vi "Save Error Logs.vi"(6 "Finish?":bool, 7 "T: no error Save":bool, 8 "error in (no error)":errorcluster, 10 "States In":string, 11 "FileName":string="Process") -> (0 "error out":errorcluster)   [LabVIEW 2021]
uses:
  TopPath/TopPath.lvlib
  <vilib>/Utility/file.llb/Write Delimited Spreadsheet (string).vi
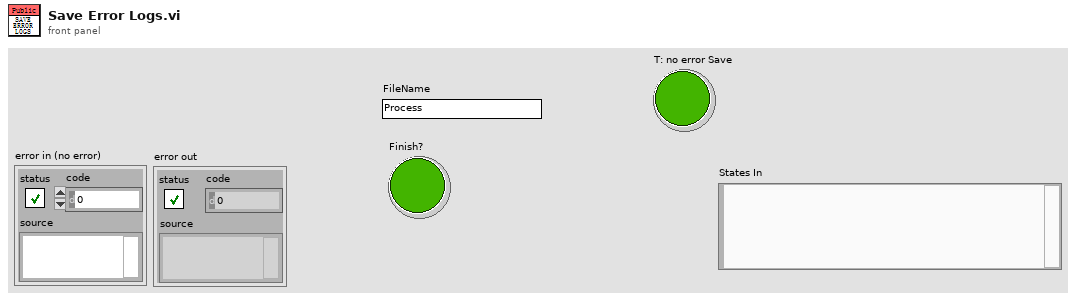
[diagram p1: front panel]
types:
  T1 = typedef "TopPath.lvlib/Top Path.ctl" = cluster{"LV Source":path, "FilePath":path, "Data":path}
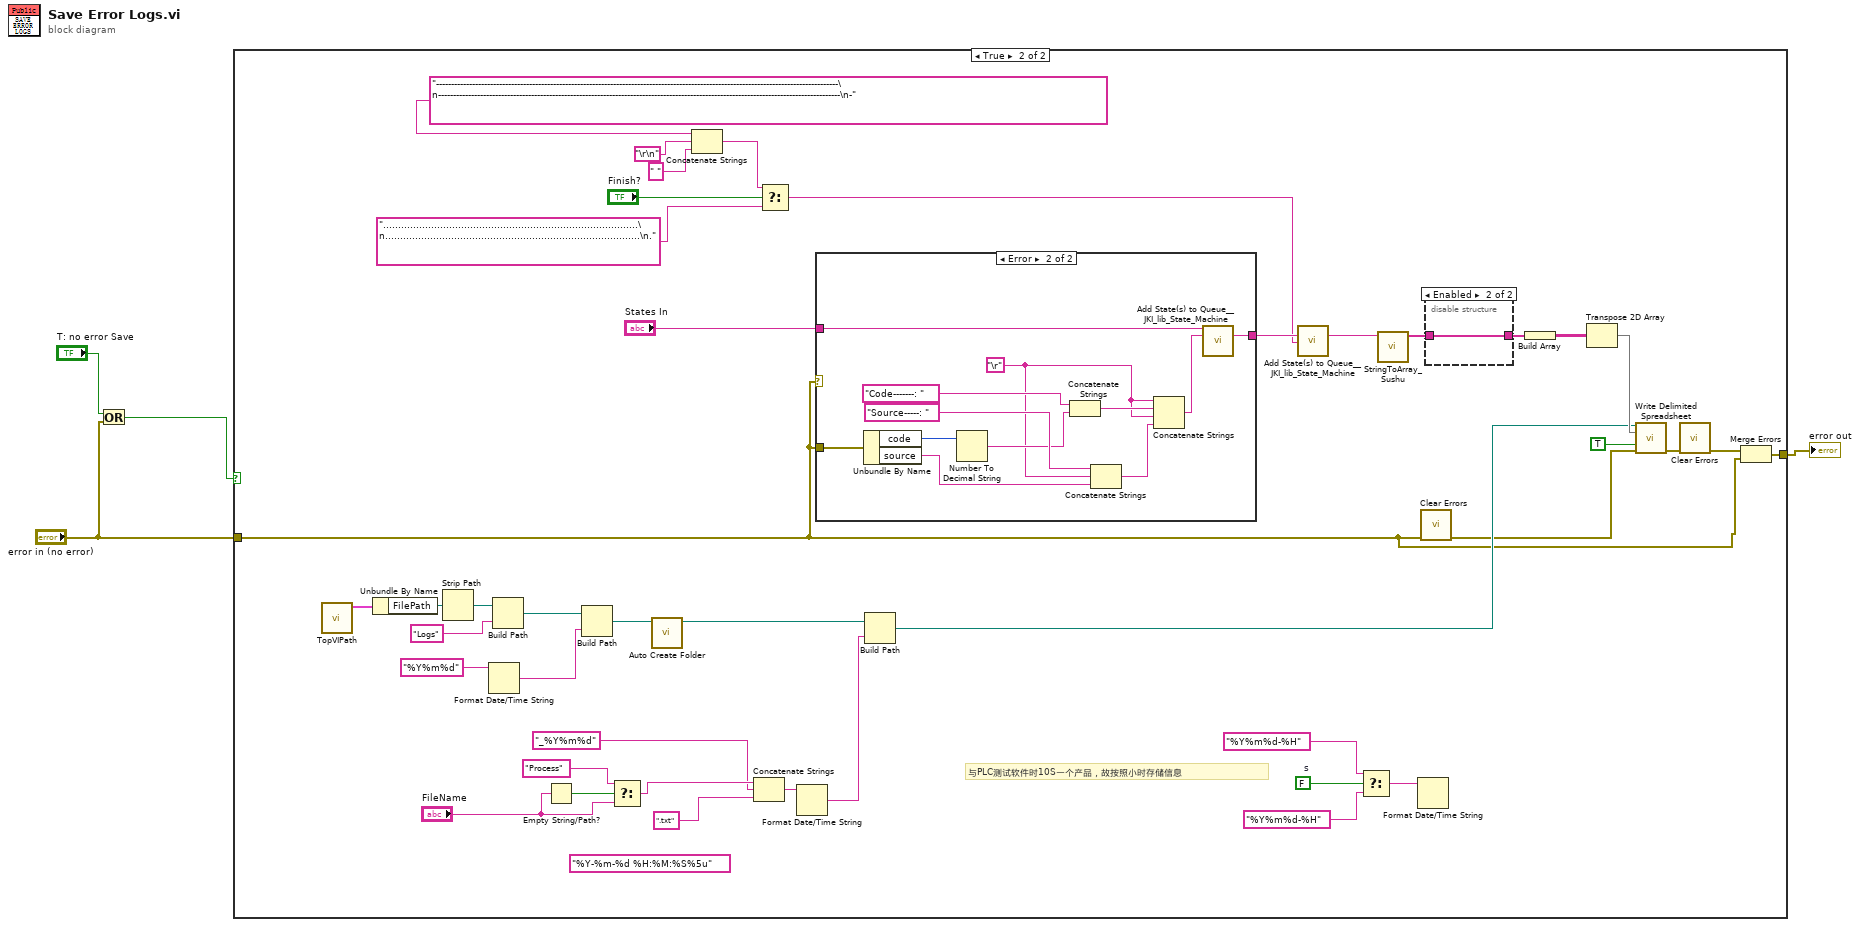
[diagram p0: block diagram]
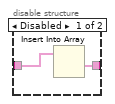
[diagram p4: hidden frame]
diagram:
  n1 = Or(x="T: no error Save", y="error in (no error)") -> (x .or. y?=w1:bool)
  n2 = case shown="True" w1 {
    tunnel: "error in (no error)" -> [w5 w7]
    tunnel: [w5 w9] -> w4
    frame False {
    }
    frame True {
      w11 = FALSE  # s
      (unwired) "%Y-%m-%d %H:%M:%S%5u" ("time format string (%c)")
      # "与PLC测试软件时10S一个产品，故按照小时存储信息"
      n3 = call "TopVIPath.vi"() -> ("TopPath"=w33:T1)  [unwired: 10 in, 1 out]
      n4 = Unbundle By Name(w33) -> ("FilePath"=w34:path)
      n5 = Strip Path(path=w34) -> (stripped path=w23:path)  [unwired: 1 out]
      n6 = Format Date/Time String(time format string (%c)="%Y%m%d") -> (date/time string=w12:string)  [unwired: 2 in]
      n7 = Build Path(base path=w23, name or relative path="Logs") -> (appended path=w15:path)
      n8 = Empty String/Path?(string/path="FileName") -> (empty?=w28:bool)
      n9 = Build Path(base path=w15, name or relative path=w12) -> (appended path=w14:path)
      n10 = Select(t="Process" ("time format string (%c)"), s=w28, f="FileName") -> (s? t:f=w25:string)
      n11 = call <userlib>:"Auto Create Folder.vi"("Folder path"=w14) -> ("Folder path"=w36:path)  [unwired: 9 in, 1 out]
      n12 = Concatenate Strings("--------------------------------------------------------------------------------------------------------------------------------------\n--------------------------------------------------------------------------------------------------------------------------------------\n-" ("string"), "\r\n", " " ("ErrorMessage")) -> (w30:string)
      n13 = Concatenate Strings(w25, "_%Y%m%d" ("time format string (%c)"), ".txt" ("string")) -> (w32:string)
      n14 = Select(t=w30, s="Finish?", f=".....................................................................................\n.....................................................................................\n.") -> (s? t:f=w19:string)
      n15 = Format Date/Time String(time format string (%c)=w32) -> (date/time string=w37:string)  [unwired: 2 in]
      n16 = case shown="Error" w7 {
        tunnel: w7 -> [_ w54]
        tunnel: [w48 w51] -> w20
        tunnel: "States In" -> [w48 w52]
        frame No Error {
        }
        frame Error {
          w49 = "\r"
          n17 = Unbundle By Name(w54) -> ("code"=w55:i32, "source"=w50:string)
          n18 = Number To Decimal String(number=w55) -> (decimal integer string=w57:string)  [unwired: 1 in]
          n19 = Concatenate Strings("Code-------: " ("string"), w57) -> (w59:string)
          n20 = Concatenate Strings("Source-----: " ("string"), w49, w50) -> (w60:string)
          n21 = Concatenate Strings(w49, w59, w49, w60) -> (w53:string)
          n22 = call <vilib>:"Add State(s) to Queue__JKI_lib_State_Machine.vi"("State(s) in Front (\"\")"=w52, "State(s) in (\"\")"=w53) -> ("States Out"=w51:string)  [unwired: 13 in]
        }
      }
      n23 = Build Path(base path=w36, name or relative path=w37) -> (appended path=w38:path)
      n24 = call <vilib>:"Add State(s) to Queue__JKI_lib_State_Machine.vi"("State(s) in (\"\")"=w20, "State(s) at Back (\"\")"=w19) -> ("States Out"=w21:string)  [unwired: 13 in]
      n25 = Select(t="%Y%m%d-%H" ("time format string (%c)"), s=w11, f="%Y%m%d-%H" ("time format string (%c)")) -> (s? t:f=w17:string)
      n26 = call <userlib>:"StringToArray_Sushu.vi"("State Queue"=w21) -> ("Array"=w42:string[])  [unwired: 7 in, 3 out]
      n27 = Format Date/Time String(time format string (%c)=w17) -> ()  [unwired: 2 in, 1 out]
      n28 = call <vilib>:"Clear Errors.vi"("error in (no error)"=w7) -> ("error out"=w8:errorcluster)  [unwired: 5 in, 1 out]
      n29 = disable-structure shown="Enabled" {
        disable-tunnel: [w62 w63] -> w43
        disable-tunnel: w42 -> [w61 w63]
        frame Disabled {
          n30 = Insert Into Array(array=w61) -> (w62:string[])  [unwired: 2 in]
        }
        frame Enabled {
        }
      }
      n31 = Build Array(w43) -> (w40:string[][])
      n32 = Transpose 2D Array(2D array=w40) -> (transposed array=w41:string[][])
      n33 = call-poly <vilib>:"Write Delimited Spreadsheet.vi"("file path (dialog if empty)"=w38, "2D data"=w41, "append to file? (new file:F)"=TRUE ("append to file? (F)"), "error in (no error)"=w8) -> ("error out"=w46:errorcluster)  [unwired: 10 in, 1 out]
      n34 = call <vilib>:"Clear Errors.vi"("error in (no error)"=w46) -> ("error out"=w6:errorcluster)  [unwired: 5 in, 1 out]
      n35 = Merge Errors(w6, w7) -> (w9:errorcluster)
    }
  }
  "error out" <- w4
